vi "motor number to motor cluster number.vi"(1 "Motor number":u16) -> (0 "number in cluster":u16)   [LabVIEW 2011]
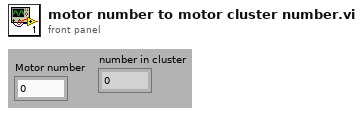
[diagram p1: front panel]
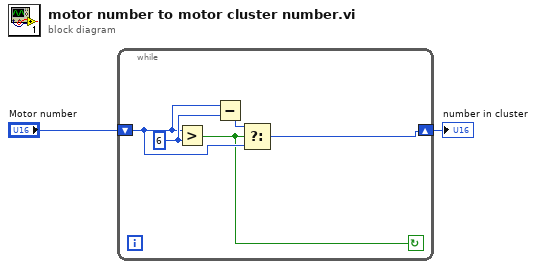
[diagram p0: block diagram]
diagram:
  n1 = while {
    shift-right: [w4] -> w1
    shift-left: "Motor number" -> [w5]
    stop <- w3 continue-if-true
    w7 = u16 6 ("y")
    n2 = Greater?(x=w5, y=w7) -> (0:w3:bool)
    n3 = Subtract(x=w5, y=w7) -> (x-y=w6:u16)
    n4 = Select(t=w6, s=w3, f=w5) -> (s? t:f=w4:u16)
  }
  "number in cluster" <- w1
